vi "DataXML setAttribute.vi"(5 "attr_value":string, 7 "attr_name":string, 8 "error in (no error)":errorcluster, 10 "target node in":refnum<k20>, 11 "DataXML in":refnum<class "DataXML.lvclass">) -> (0 "error out":errorcluster, 2 "target node out":refnum<k20>, 3 "DataXML out":refnum<class "DataXML.lvclass">)   [LabVIEW 2018, in "DataXML.lvclass"]
uses:
  DataXML.lvclass
  <resource>/objmgr/DOMUserDefRef.rc
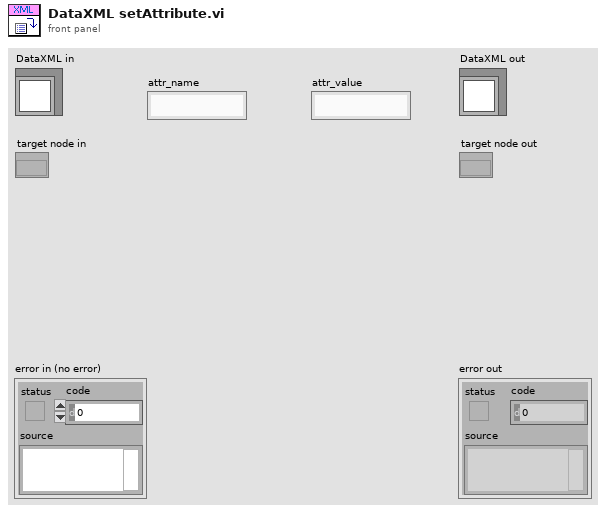
[diagram p1: front panel]
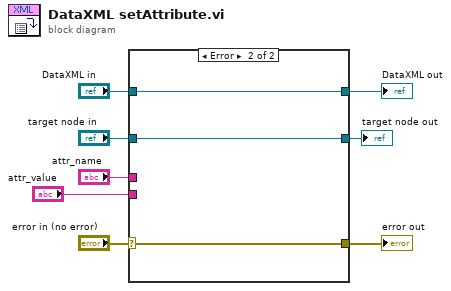
[diagram p0: block diagram]
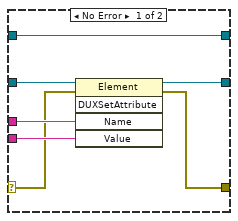
[diagram p2: hidden frame]
diagram:
  n1 = case shown="Error" "error in (no error)" {
    selector: "error in (no error)" -> [w11 w18]
    tunnel: [w10 w18] -> w7
    tunnel: [w15 w17] -> w5
    tunnel: "DataXML in" -> [w15 w17]
    tunnel: "target node in" -> [w14 w16]
    tunnel: "attr_name" -> [w13 _]
    tunnel: "attr_value" -> [w12 _]
    tunnel: [w9 w16] -> w1
    frame No Error {
      n2 = invoke class="Element" method="DUXSetAttribute"(reference=w14, error in=w11, "Name"=w13, "Value"=w12) -> (reference out=w9:refnum<k20>, error out=w10:errorcluster)  [unwired: 1 in, 3 out]
    }
    frame Error {
    }
  }
  "error out" <- w7
  "DataXML out" <- w5
  "target node out" <- w1
